vi "InsertIntoShortcutMenu.vi"(8 "error in":errorcluster, 9 "menu ref in":refnum<k9>, 11 "System in":refnum<class "System.lvclass">) -> (0 "error out":errorcluster, 1 "menu ref out":refnum<k9>, 3 "System out":refnum<class "System.lvclass">)   [LabVIEW 2025, in "System.lvlib" / "System.lvclass"]
doc: "Allows children to insert menu items without overriding ShortcutMenu.vi entirely. By default, called before Add/Remove.Copyright 2017 National Instruments Corporation\n\nLicensed under the Apache License, Version 2.0 (the \"License\"); you may not use this file except in compliance with the License. You may obtain a copy of the License at http://www.apache.org/licenses/LICENSE-2.0\nUnless required by applicable law or agreed to in writing, software distributed under the License is distributed on an \"AS IS\" BASIS, WITHOUT WARRANTIES OR CONDITIONS OF ANY KIND, either express or implied. See the License for the specific language governing permissions and limitations under the License."
uses:
  System.lvclass
  Users/Public/Documents/Sandia National Labs/TSS Plugin/CEF.lvlibp/Node/ReadChildren.vi
  Users/Public/Documents/Sandia National Labs/TSS Plugin/CEF.lvlibp/Node/ReadNodeClass.vi
  Users/Public/Documents/Sandia National Labs/TSS Plugin/CEF.lvlibp/Node/CEF_Node.lvclass
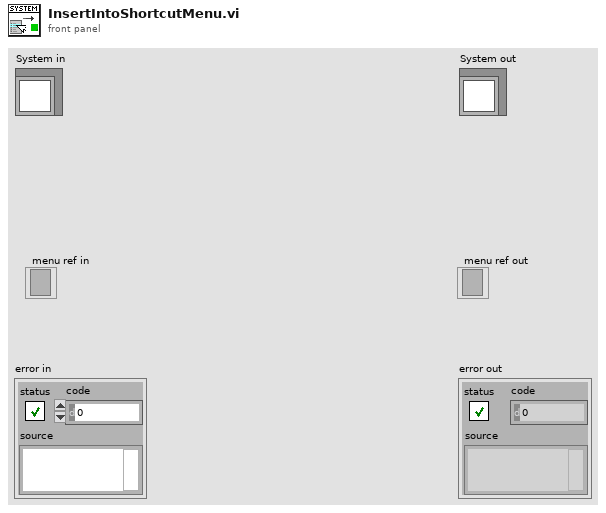
[diagram p1: front panel]
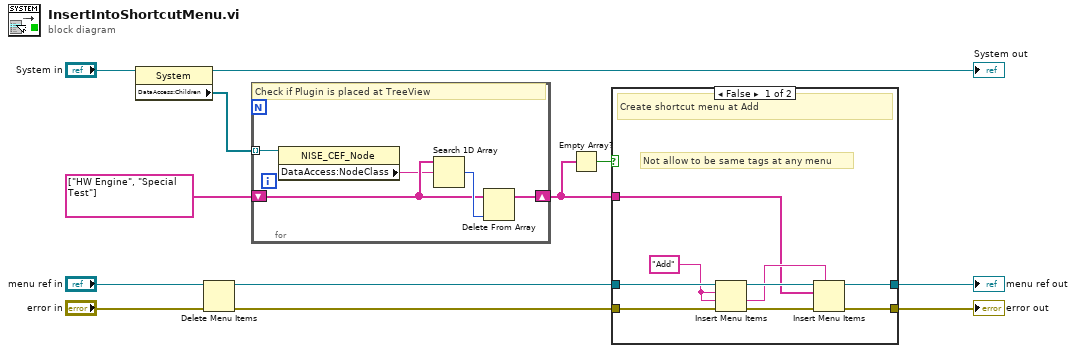
[diagram p0: block diagram]
diagram:
  n1 = property class="System"(reference="System in") -> (reference out=→"System out":refnum<class "System.lvclass">, "DataAccess:Children"=w10:refnum<data-value>[])  [unwired: 1 in, 1 out]
  n2 = Delete Menu Items(6:"error in", 9:"menu ref in") -> (0:w3:errorcluster, 3:w4:refnum<k9>)  [unwired: 2 in]
  n3 = for {
    tunnel: w10 -> [w14] mode=indexing
    shift-right: [w15] -> w6
    shift-left: string[] ["HW Engine", "Special Test"] -> [w16]
    # "Check if Plugin is placed at TreeView"
    n4 = property class="NISE_CEF_Node"(reference=w14) -> ("DataAccess:NodeClass"=w13:string)  [unwired: 1 in, 2 out]
    n5 = Search 1D Array(1D array=w16, element=w13) -> (index of element=w17:i32)  [unwired: 1 in]
    n6 = Delete From Array(array=w16, index=w17) -> (array with subset deleted=w15:string[])  [unwired: 1 in, 1 out]
  }
  n7 = Empty Array?(array=w6) -> (empty?=w5:bool)
  n8 = case shown="False" w5 {
    tunnel: w3 -> [w26 w28]
    tunnel: [w19 w27] -> w2
    tunnel: w4 -> [w25 w27]
    tunnel: [w20 w28] -> w1
    tunnel: w6 -> [w18 _]
    frame False {
      w22 = "Add"
      # "Not allow to be same tags at any menu"
      # "Create shortcut menu at Add"
      n9 = Insert Menu Items(6:w26, 7:w22, 8:w22, 9:w25) -> (0:w23:errorcluster, 1:w21:string, 3:w24:refnum<k9>)  [unwired: 2 in]
      n10 = Insert Menu Items(5:w21, 6:w23, 8:w18, 9:w24) -> (0:w20:errorcluster, 3:w19:refnum<k9>)  [unwired: 2 in, 1 out]
    }
    frame True {
      # "If all plugins are in TreeView, shortcut menu does not be showed up"
    }
  }
  "error out" <- w1
  "menu ref out" <- w2
